vi "__updateConfiguration.vi"(8 "error in (no error)":errorcluster, 11 "Room-API in":refnum<class "Room-API.lvclass">) -> (0 "error out":errorcluster, 3 "Room-API out":refnum<class "Room-API.lvclass">)   [LabVIEW 2020, in "Room-API.lvclass"]
uses:
  Room-API.lvclass
  Room-API.lvclass/Room-API.ctl
  7ec09309-529f-4387-ae0a-b5679fbe9b57.vi
  <vilib>/JDP Science/JSONtext/Variant to JSON Text.vi
  <vilib>/JDP Science/JSONtext/support/Format JSON Object.vi
  <vilib>/JDP Science/JSONtext/JSONtext.lvlib
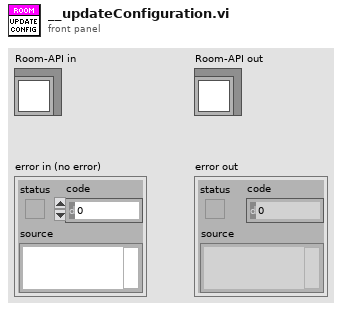
[diagram p1: front panel]
types:
  T1 = enum16{"open", "replace", "create", "open or create", "replace or create", "replace or create with confirmation"}
  T2 = typedef "Room-API.lvclass/Single Room.ctl" = cluster{"name":string, "temperature_humidity":string[], "bond":string[], "hue":string[]}
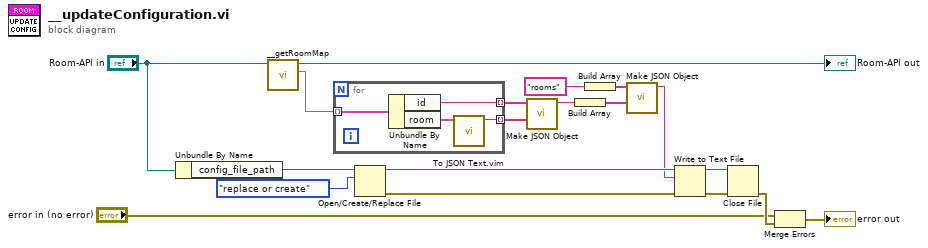
[diagram p0: block diagram]
diagram:
  n1 = Unbundle By Name("Room-API in") -> ("config_file_path"=w10:path)
  n2 = call "__getRoomMap.vi"("Room-API in"="Room-API in") -> ("room_map"=w17:map{string, T2}, "Room-API out"=→"Room-API out":refnum<class "Room-API.lvclass">)  [unwired: 9 in]
  n3 = for {
    tunnel: w17 -> [w23] mode=indexing
    tunnel: [w21] -> w16 mode=indexing
    tunnel: [w20] -> w15 mode=indexing
    n4 = Unbundle By Name(w23) -> ("id"=w21:string, "room"=w22:T2)
    n5 = call "To JSON Text.vim"("Anything"=w22) -> ("<JSON>"=w20:string)  [unwired: 9 in, 1 out]
  }
  n6 = Open/Create/Replace File(file path (use dialog)=w10, operation (0:open)=T1."replace or create") -> (refnum out=w8:refnum<file>, error out=w7:errorcluster)  [unwired: 4 in, 1 out]
  n7 = call <vilib>:"Make JSON Object.vi"("JSON Items"=w15, "Item Names"=w16) -> ("<JSON>"=w13:string)  [unwired: 8 in, 1 out]
  n8 = Build Array(w13) -> (w12:string[])
  n9 = Build Array("rooms") -> (w11:string[])
  n10 = call <vilib>:"Make JSON Object.vi"("JSON Items"=w12, "Item Names"=w11) -> ("<JSON>"=w6:string)  [unwired: 8 in, 1 out]
  n11 = Write to Text File(file (use dialog)=w8, text=w6, error in=w7) -> (refnum out=w5:refnum<file>, error out=w4:errorcluster)  [unwired: 1 in, 1 out]
  n12 = Close File(refnum=w5, error in=w4) -> (error out=w3:errorcluster)  [unwired: 1 out]
  n13 = Merge Errors("error in (no error)", w3) -> (→"error out":errorcluster)
